vi "TAMANHO-SERVER 2.vi"() -> ()   [LabVIEW 2019]
panel:
  in  "stop":bool
  in  "size":i32
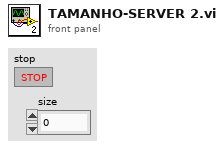
[diagram p1: front panel]
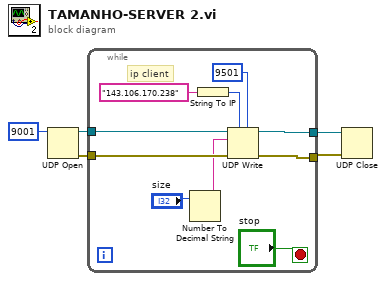
[diagram p0: block diagram]
diagram:
  n1 = UDP Open(11:u16 9001 ("port")) -> (port=w4:refnum<k16>, 0:w2:errorcluster)  [unwired: 4 in, 1 out]
  n2 = while {
    tunnel: w4 -> [w15]
    tunnel: [w14] -> w3
    tunnel: w2 -> [w13]
    tunnel: [w12] -> w1
    stop <- "stop" stop-if-true
    # "ip client"
    n3 = Number To Decimal String(number="size") -> (decimal integer string=w7:string)  [unwired: 1 in]
    n4 = String To IP(1:"143.106.170.238" ("name")) -> (0:w11:u32)
    n5 = UDP Write(address=w11, port or service name=u16 9501, connection ID=w15, data in=w7, 8:w13) -> (error out=w12:errorcluster, 3:w14:refnum<k16>)  [unwired: 1 in]
  }
  n6 = UDP Close(connection ID=w3, 8:w1) -> ()  [unwired: 2 out]
